vi "Init AO DAQ v2.vi"(8 "error in":errorcluster, 10 "DAQChan[]":T1[](array[typedef])) -> (0 "error out":errorcluster, 3 "AO TaskRefs":refnum<k21>[](array[refnum]))   [LabVIEW 2017]
doc: "Developed by Kevin Thompson\nThompson Engineering, LLC\nkevin@thompsonengineering.net"
uses:
  Analog DAQChan--cluster.ctl
  AI InstrType--enum.ctl
  <vilib>/DAQmx/create/channels.llb/DAQmx Create Channel (AO-Voltage-Basic).vi
  <vilib>/DAQmx/create/channels.llb/DAQmx Create Channel (AO-Current-Basic).vi
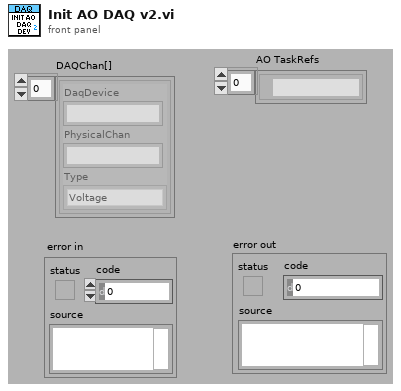
[diagram p1: front panel]
types:
  T1 = typedef "Analog DAQChan--cluster.ctl" = cluster{"DaqDevice":string, "PhysicalChan":string, "Type":T2}
  T2 = typedef "AI InstrType--enum.ctl" = enum16{"Voltage", "Current"}
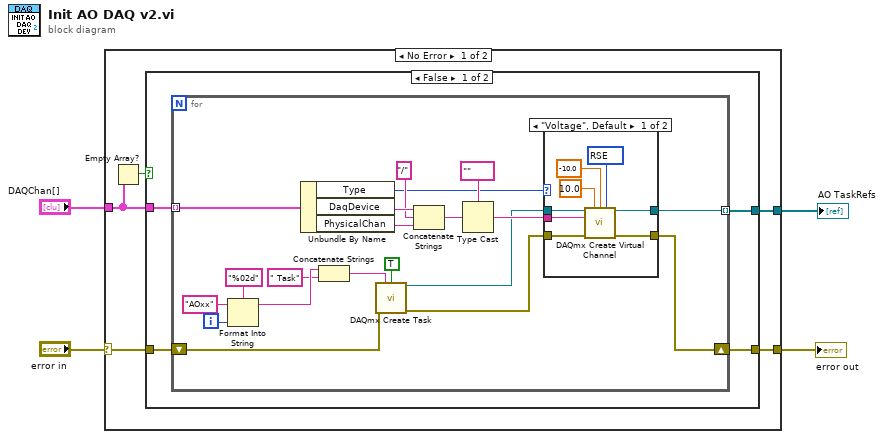
[diagram p0: block diagram]
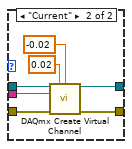
[diagram p2: hidden frame]
diagram:
  n1 = case shown="No Error" "error in" {
    selector: "error in" -> [w7 w50]
    tunnel: "DAQChan[]" -> [w5 _]
    tunnel: [w9 w50] -> w3
    tunnel: [w8 _] -> w1
    frame No Error {
      n2 = Empty Array?(array=w5) -> (empty?=w6:bool)
      n3 = case shown="False" w6 {
        tunnel: w5 -> [w13 _]
        tunnel: [w12 w49] -> w9
        tunnel: [w11 _] -> w8
        tunnel: w7 -> [w10 w49]
        frame False {
          n4 = for {
            tunnel: w13 -> [w33] mode=indexing
            shift-right: [w25] -> w12
            shift-left: w10 -> [w17]
            tunnel: [w14] -> w11 mode=indexing
            i -> [w18]
            n5 = Format Into String(format string="%02d", initial string="AOxx", w18) -> (resulting string=w24:string)  [unwired: 1 in, 1 out]
            n6 = Unbundle By Name(w33) -> ("Type"=w26:T2, "DaqDevice"=w32:string, "PhysicalChan"=w30:string)
            n7 = Concatenate Strings(w24, " Task" ("string")) -> (w23:string)
            n8 = call <vilib>:"DAQmx Create Task.vi"("new task name"=w23, "auto cleanup"=TRUE, "error in"=w17) -> ("task out"=w15:refnum<k21>, "error out"=w16:errorcluster)  [unwired: 11 in]
            n9 = Concatenate Strings(w32, "/", w30) -> (w28:string)
            n10 = Type Cast(type=tag "" ("PhysChan"), x=w28) -> (*(type *) &x=w27:tag)
            n11 = case shown="\"Voltage\", Default" w26 {
              tunnel: w27 -> [w41 w48]
              tunnel: w16 -> [w38 w45]
              tunnel: [w37 w44] -> w25
              tunnel: [w39 w46] -> w14
              tunnel: w15 -> [w40 w47]
              frame "Voltage", Default {
                w34 = 10083 items=["Default"=-1, "RSE"=10083, "Differential"=10106, "Pseudodifferential"=12529] ("output terminal configuration")
                n12 = call-poly <vilib>:"DAQmx Create Virtual Channel.vi"("task in"=w40, "maximum value"=10.0, "minimum value"=-10.0, "output terminal configuration"=w34, "physical channels"=w41, "error in"=w38) -> ("task out"=w39:refnum<k21>, "error out"=w37:errorcluster)  [unwired: 8 in]
              }
              frame "Current" {
                n13 = call-poly <vilib>:"DAQmx Create Virtual Channel.vi"("task in"=w47, "maximum value"=0.02, "minimum value"=-0.02, "physical channels"=w48, "error in"=w45) -> ("task out"=w46:refnum<k21>, "error out"=w44:errorcluster)  [unwired: 9 in]
              }
            }
          }
        }
        frame True {
        }
      }
    }
    frame Error {
    }
  }
  "error out" <- w3
  "AO TaskRefs" <- w1
